vi "Current Field v0.80.vi"(2 "error in (no error)":errorcluster) -> (0 "error out":errorcluster, 1 "Field Output":dbl format="%.2f")   [LabVIEW 2019]
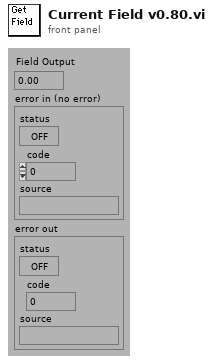
[diagram p1: front panel]
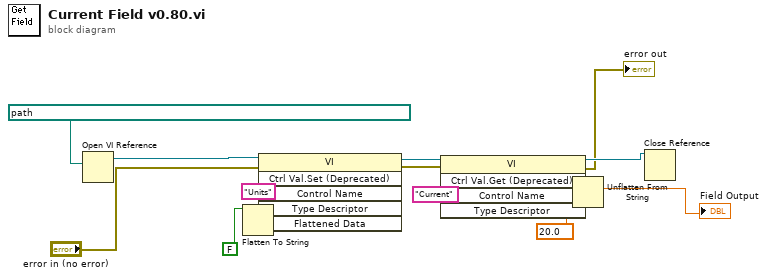
[diagram p0: block diagram]
diagram:
  n1 = Open VI Reference(vi path=path "/Optics2Mac/xwei Work/NML Data Acq/Serial Instruments/PS ƒ/PS Control") -> (vi reference=w2:refnum<vi>)  [unwired: 5 in, 1 out]
  n2 = Flatten To String(anything=FALSE ("Wait until done")) -> (data string=w14:string, type string=w13:i16[])  [unwired: 3 in, 1 out]
  n3 = invoke class="VI" method="Ctrl Val.Set (Deprecated)"(reference=w2, error in="error in (no error)", "Control Name"="Units", "Type Descriptor"=w13, "Flattened Data"=w14) -> (reference out=w8:refnum<vi>, error out=w4:errorcluster)  [unwired: 1 in, 4 out]
  n4 = invoke class="VI" method="Ctrl Val.Get (Deprecated)"(reference=w8, error in=w4, "Control Name"="Current") -> (reference out=w6:refnum<vi>, error out=→"error out":errorcluster, "Get Control Value"=w9:string)  [unwired: 2 in, 2 out]
  n5 = Unflatten From String(type=20.0 ("Desired Field (T)"), binary string=w9) -> (value=→"Field Output":dbl)  [unwired: 3 in, 2 out]
  n6 = Close Reference(reference=w6) -> ()  [unwired: 1 in, 1 out]
